vi "request.vi"(7 "request":string, 8 "error in (no error)":errorcluster, 10 "Parameter":variant, 11 "TaskRef in":refnum<vi>) -> (0 "error IO":errorcluster, 3 "TaskRef out":refnum<vi>)   [LabVIEW 2015, in "pdbm_task_route.lvlib"]
uses:
  pdbm_task_route.lvlib
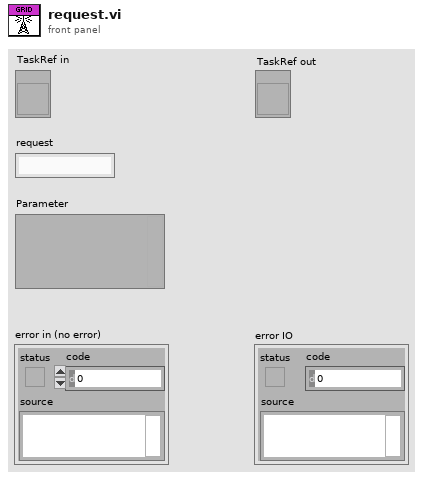
[diagram p1: front panel]
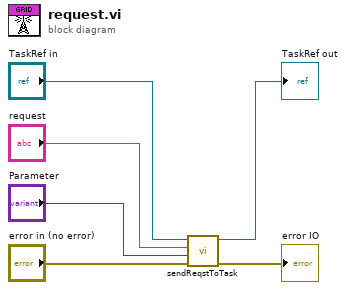
[diagram p0: block diagram]
diagram:
  n1 = call "sendReqstToTask.vi"("error in (no error)"="error in (no error)", "Parameter"="Parameter", "request"="request", "TaskRef in"="TaskRef in") -> ("error IO"=→"error IO":errorcluster, "TaskRef out"=→"TaskRef out":refnum<vi>)  [unwired: 6 in]
